vi "Read AB Tovey Serial Settings.vi"(8 "error in (no error)":errorcluster, 11 "Boot Loader in":refnum<class "Boot Loader.lvclass">) -> (0 "error out":errorcluster, 2 "Serial":T1={"Serial Protocol"=enum."RS485", "Protocol Parameters"={"VISA resource name"="", "Baud Rate"=9600, "Data Bits"=8, "Parity"=enum."None", "Flow Control"=0, "Stop Bits"=10, "Timeout (ms)"=10000}, "Serial Message Parameters"={"Byte Count"=200, "Enable Termination Character"=FALSE, "Termination Char"=200}} {"Serial Message Parameters"."Termination Char" format="%x"; "Protocol Parameters"."Stop Bits" items=["1.0"=10, "1.5"=15, "2.0"=20]; "Protocol Parameters"."Flow Control" items=["None", "XON/XOFF", "RTS/CTS", "XON/XOFF & RTS/CTS", "DTR/DSR", "XON/XOFF & DTR/DSR"]; "Protocol Parameters"."Data Bits" min=5 max=8 step=1}, 3 "Boot Loader out":refnum<class "Boot Loader.lvclass">)   [LabVIEW 2015, in "Boot Loader.lvclass"]
uses:
  Boot Loader.lvclass
  <userlib>/Common/SerialProtocols/Configuration/SerialConfig.ctl
  <userlib>/Common/SerialProtocols/Configuration/SerialProtocol.ctl
  <userlib>/Common/SerialProtocols/Configuration/ProtocolParameters.ctl
  <userlib>/Common/SerialProtocols/Configuration/SerialMessageParameters.ctl
  <userlib>/Common/SerialProtocols/SerialProtocols.lvlib
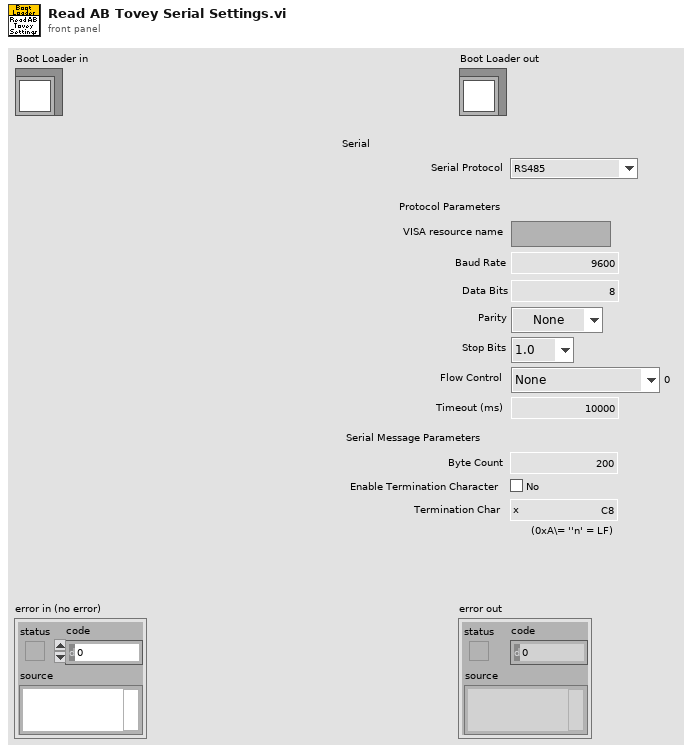
[diagram p1: front panel]
types:
  T1 = typedef "SerialProtocols.lvlib/SerialConfig.ctl" = cluster{"Serial Protocol":T2, "Protocol Parameters":T3, "Serial Message Parameters":T4}
  T2 = typedef "SerialProtocols.lvlib/SerialProtocol.ctl" = enum16{"RS232", "RS485", "SerialSimulator"}
  T3 = typedef "SerialProtocols.lvlib/ProtocolParameters.ctl" = cluster{"VISA resource name":refnum<visa-resource-name>, "Baud Rate":u32, "Data Bits":u16, "Parity":enum16{"None", "Odd", "Even", "Mark", "Space"}, "Flow Control":u16, "Stop Bits":u16, "Timeout (ms)":u32}
  T4 = typedef "SerialProtocols.lvlib/SerialMessageParameters.ctl" = cluster{"Byte Count":u32, "Enable Termination Character":bool, "Termination Char":u8}
  T5 = typedef "FAMT Typedefs.lvlib/Serial Settings.ctl" = cluster{"Baud Rate":u32, "Data Bits":u16, "Parity":enum16{"None", "Odd", "Even", "Mark", "Space"}, "Flow Control":u16, "Stop Bits":u16, "Timeout (ms)":u32, "Byte Count":u32, "Enable Termination Character":bool, "Termination Char":u8}
  T6 = typedef "FAMT Typedefs.lvlib/Connection Settings.ctl" = cluster{"Pressure Servo Valve 1 DAC":u8, "Pressure Servo Valve 2 DAC":u8, "Flow Control Valve DAC":u8, "Load Cell ADC":u8, "FC1 ILC Port":refnum<visa-resource-name>, "FC2 ILC Port":refnum<visa-resource-name>, "Tovey A-B Port":refnum<visa-resource-name>, "Tovey C-D Port":refnum<visa-resource-name>, "Tovey E-F Port":refnum<visa-resource-name>, "FC1 ILC Protocol":T2, "FC2 ILC Protocol":T2, "Tovey A-B Protocol":T2, "Tovey C-D Protocol":T2, "Tovey E-F Protocol":T2, "Tovey A-B Address":u8, "Tovey C-D Address":u8, "Tovey E-F Address":u8}
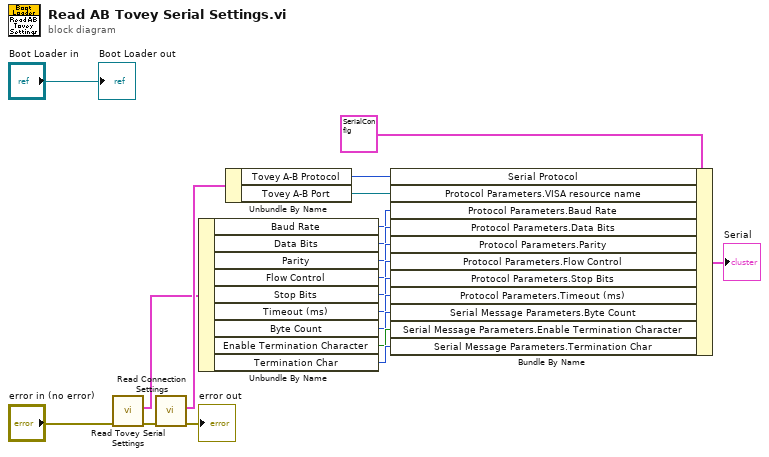
[diagram p0: block diagram]
diagram:
  n1 = call "Read Tovey Serial Settings.vi"("error in (no error)"="error in (no error)") -> ("error out"=w4:errorcluster, "Serial Settings"=w3:T5)  [unwired: 8 in, 1 out]
  n2 = call "Read Connection Settings.vi"("error in (no error)"=w4) -> ("error out"=→"error out":errorcluster, "Connection Settings"=w8:T6)  [unwired: 8 in, 1 out]
  n3 = Unbundle By Name(w3) -> ("Baud Rate"=w10:u32, "Data Bits"=w11:u16, "Parity"=w12:enum16{"None", "Odd", "Even", "Mark", "Space"}, "Flow Control"=w13:u16, "Stop Bits"=w14:u16, "Timeout (ms)"=w15:u32, "Byte Count"=w16:u32, "Enable Termination Character"=w17:bool, "Termination Char"=w18:u8)
  n4 = Unbundle By Name(w8) -> ("Tovey A-B Protocol"=w7:T2, "Tovey A-B Port"=w6:refnum<visa-resource-name>)
  n5 = Bundle By Name(cluster=T1 {"Serial Protocol"=enum."RS485", "Protocol Parameters"={"VISA resource name"="", "Baud Rate"=9600, "Data Bits"=8, "Parity"=enum."None", "Flow Control"=0, "Stop Bits"=10, "Timeout (ms)"=10000}, "Serial Message Parameters"={"Byte Count"=200, "Enable Termination Character"=FALSE, "Termination Char"=200}} ("Serial"), "Serial Protocol"=w7, "Protocol Parameters.VISA resource name"=w6, "Protocol Parameters.Baud Rate"=w10, "Protocol Parameters.Data Bits"=w11, "Protocol Parameters.Parity"=w12, "Protocol Parameters.Flow Control"=w13, "Protocol Parameters.Stop Bits"=w14, "Protocol Parameters.Timeout (ms)"=w15, "Serial Message Parameters.Byte Count"=w16, "Serial Message Parameters.Enable Termination Character"=w17, "Serial Message Parameters.Termination Char"=w18) -> (→"Serial":T1)
  "Boot Loader out" <- "Boot Loader in"
